vi "Motor control with speed PID.vi"(6 "Motor Connectors":T4={"Enable"="ConnectorB/DIO0", "Input 1"="ConnectorA/DIO1", "Input 2"="ConnectorA/DIO2", "Tach 1"="ConnectorB/DIO8", "Tach 2"="ConnectorB/DIO9"}, 7 "Control":T3={"Motor PWM Control"={"Pulse Lenght DIO3"=10000, "Pulse Period 3"=20000, "Angle"=0}, "stop"=FALSE, "Update Insides Values"=FALSE, "Position Reset"=FALSE}) -> (1 "Speed Output":T5, 2 "Position Output":T6, 3 "Inside values":T7)   [LabVIEW 2013]
uses:
  <vilib>/eio/EIONode/EIONode.xnode
  <vilib>/rvi/eio/common/nirviEmuTemplateMethod_errors.vi
panel:
  in  "Encoder Intputs Motor 3":T1
  in  "Encoder Intputs Motor 2":T1
  out "Incrementation/Decrementation Motor 3":bool
  out "Movement Motor 3":bool
  out "Incrementation/Decrementation Motor 2":bool
  out "Movement Motor 2":bool
  in  "Encoder Intputs Motor 1":T1
  out "Movement Motor 1":bool
  out "Incrementation/Decrementation Motor 1":bool
  in  "Motor Values":T2
  in  "Inside values Motor 3":cluster{"Pulse Lenght":i32, "Angle":i32}
  in  "Inside values Motor 2":cluster{"Pulse Lenght":i32, "Angle":i32}
  in  "Inside values Motor 1":cluster{"Pulse Lenght":i32, "Angle":i32}
  out "Position Reset":bool
  out "Velocity (Counts/Interval)":i32
  out "Degree (absolute)":i32
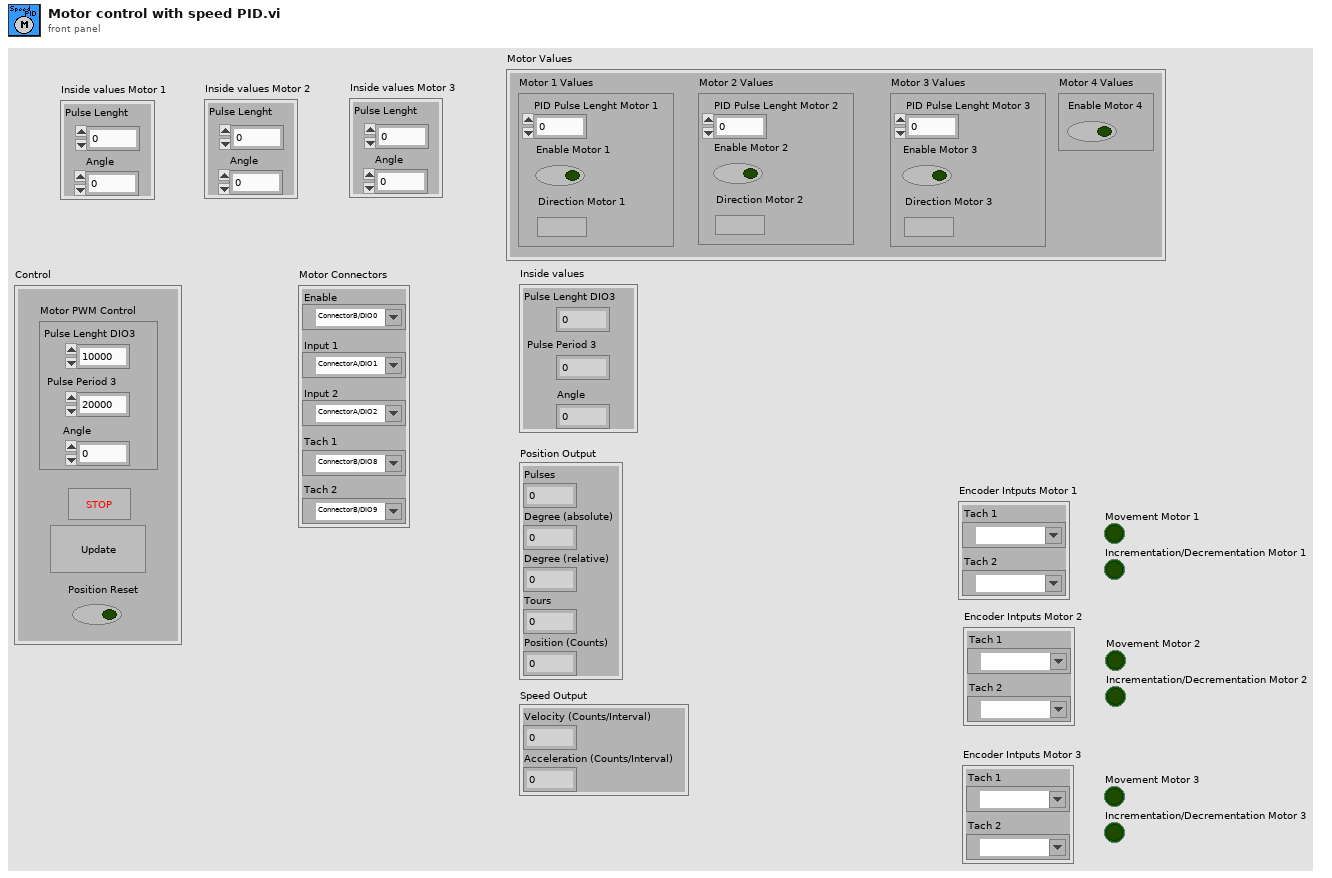
[diagram p1: front panel]
types:
  T1 = cluster{"Tach 2":refnum<k21>, "Tach 1":refnum<k21>}
  T2 = cluster{"Motor 1 Values":cluster{"PID Pulse Lenght Motor 1":i16, "Enable Motor 1":bool, "Direction Motor 1":bool}, "Motor 2 Values":cluster{"PID Pulse Lenght Motor 2":i16, "Enable Motor 2":bool, "Direction Motor 2":bool}, "Motor 3 Values":cluster{"PID Pulse Lenght Motor 3":i16, "Enable Motor 3":bool, "Direction Motor 3":bool}, "Motor 4 Values":cluster{"Enable Motor 4":bool}}
  T3 = cluster{"Motor PWM Control":cluster{"Pulse Lenght DIO3":i32, "Pulse Period 3":i32, "Angle":i32}, "stop":bool, "Update Insides Values":bool, "Position Reset":bool}
  T4 = cluster{"Enable":refnum<k21>, "Input 1":refnum<k21>, "Input 2":refnum<k21>, "Tach 1":refnum<k21>, "Tach 2":refnum<k21>}
  T5 = cluster{"Velocity (Counts/Interval)":i32, "Acceleration (Counts/Interval)":i32}
  T6 = cluster{"Pulses":i32, "Degree (absolute)":i32, "Degree (relative)":i32, "Tours":i32, "Position (Counts)":i32}
  T7 = cluster{"Pulse Lenght DIO3":i32, "Pulse Period 3":i32, "Angle":i32}
  T8 = cluster{"Velocity Interval (uSec)":i32, "I/O Tach 1":bool, "I/O Tach 2":bool, "Position (Counts)":i16, "Boolean Variable 1":bool, "Tick Count(Ticks)":u32, "Position (Counts) 2":i16, "Acceleration (Counts/Interval)":i16, "Velocity (Counts/Interval":i16}
  T9 = cluster{"PID Pulse Lenght Motor 1":i16, "Enable Motor 1":bool, "Direction Motor 1":bool}
  T10 = cluster{"PID Pulse Lenght Motor 2":i16, "Enable Motor 2":bool, "Direction Motor 2":bool}
  T11 = cluster{"PID Pulse Lenght Motor 3":i16, "Enable Motor 3":bool, "Direction Motor 3":bool}
  T12 = cluster{"Tach 1":refnum<k21>, "Tach 2":refnum<k21>}
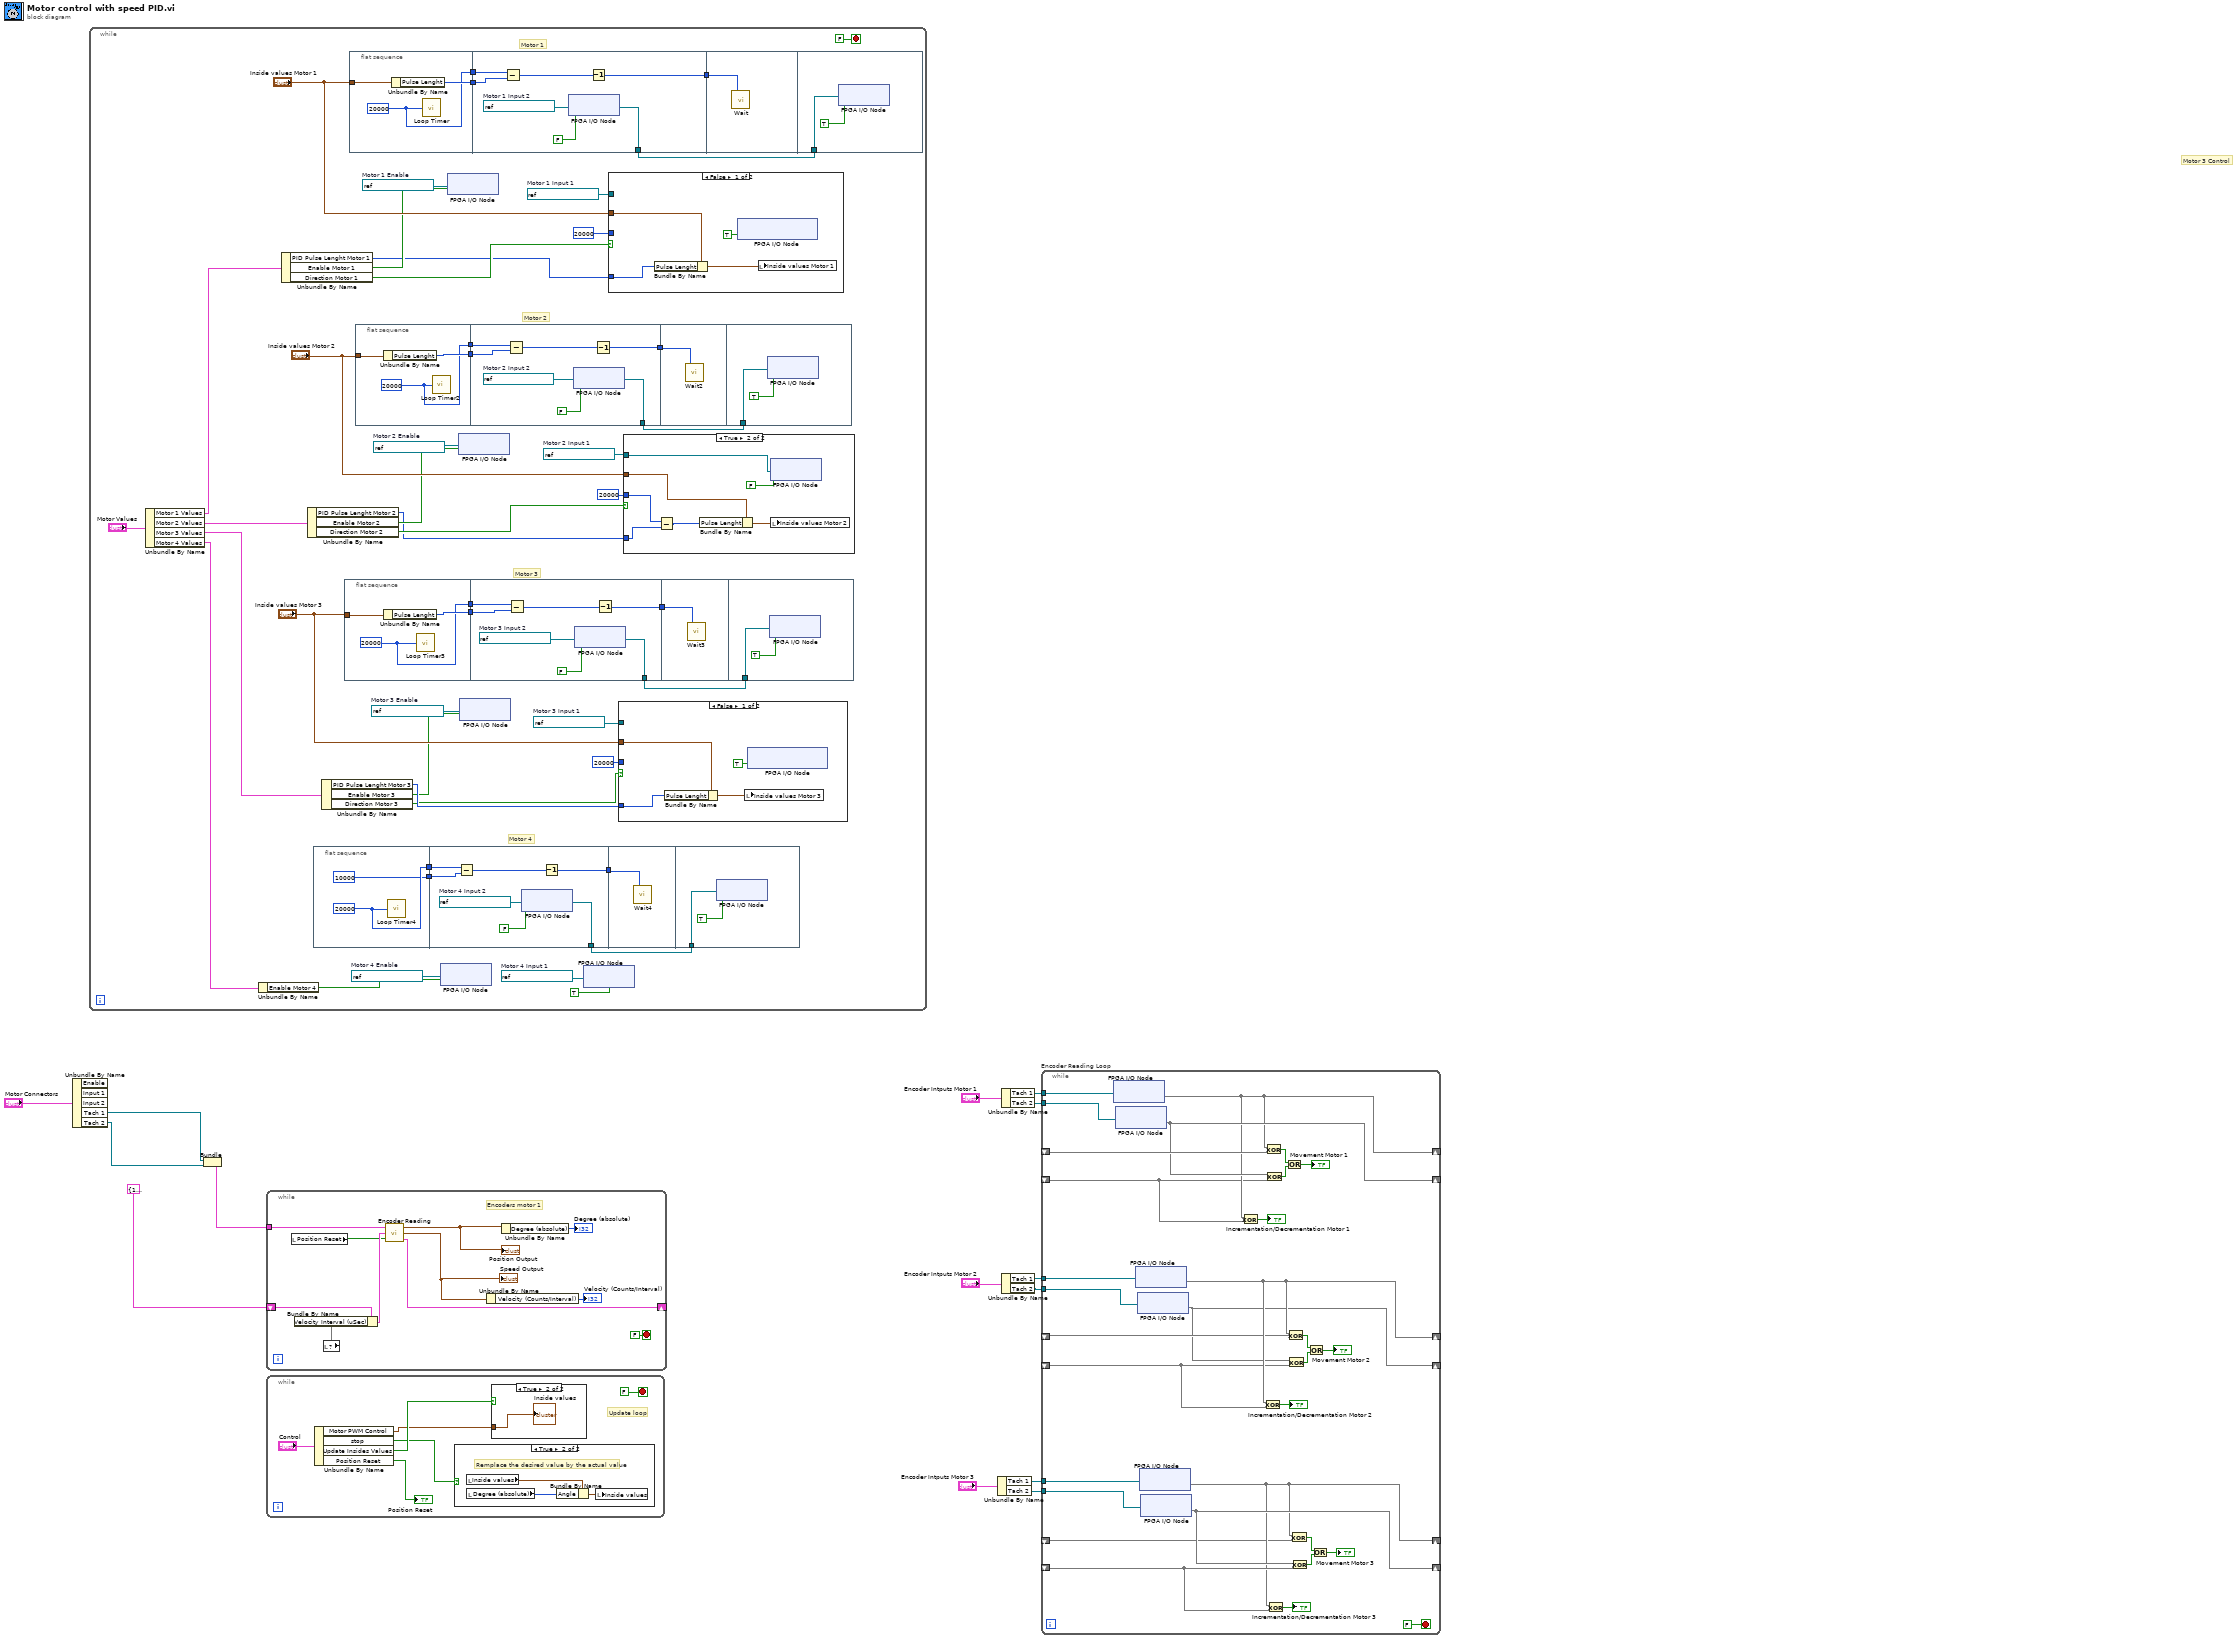
[diagram p0: block diagram]
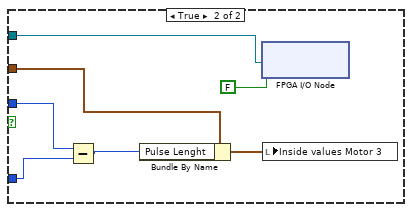
[diagram p2: hidden frame]
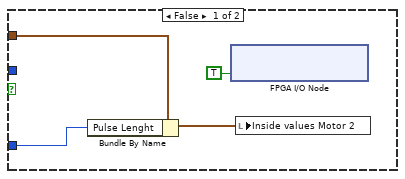
[diagram p3: hidden frame]
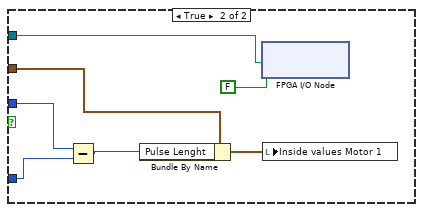
[diagram p4: hidden frame]
diagram:
  # "Motor 3 Control"
  n1 = Unbundle By Name("Motor Connectors") -> ("Tach 1"=w13:refnum<k21>, "Tach 2"=w12:refnum<k21>)  [unwired: 3 out]
  n2 = while {
    stop <- FALSE stop-if-true
    w36 = refnum<k21> "ConnectorA/DIO4"  # Motor 4 Input 1
    w38 = refnum<k21> "ConnectorA/DIO3"  # Motor 4 Enable
    w40 = refnum<k21> "ConnectorA/DIO0"  # Motor 3 Enable
    w39 = refnum<k21> "ConnectorA/DIO1"  # Motor 3 Input 1
    w41 = refnum<k21> "ConnectorB/DIO4"  # Motor 2 Input 1
    w42 = refnum<k21> "ConnectorB/DIO3"  # Motor 2 Enable
    w43 = refnum<k21> "ConnectorB/DIO1"  # Motor 1 Input 1
    w44 = refnum<k21> "ConnectorB/DIO0"  # Motor 1 Enable
    # "Motor 2"
    # "Motor 1"
    # "Motor 3"
    # "Motor 4"
    n3 = Unbundle By Name("Motor Values") -> ("Motor 1 Values"=w28:T9, "Motor 2 Values"=w24:T10, "Motor 3 Values"=w20:T11, "Motor 4 Values"=w16:cluster{"Enable Motor 4":bool})
    n4 = Unbundle By Name(w16) -> ("Enable Motor 4"=w15:bool)
    n5 = Unbundle By Name(w28) -> ("PID Pulse Lenght Motor 1"=w25:i16, "Enable Motor 1"=w27:bool, "Direction Motor 1"=w26:bool)
    n6 = Unbundle By Name(w24) -> ("PID Pulse Lenght Motor 2"=w21:i16, "Enable Motor 2"=w23:bool, "Direction Motor 2"=w22:bool)
    n7 = flat-sequence {
      tunnel: [w63] -> w48
      tunnel: [i16 10000] -> w47
      tunnel: [w70] -> w46
      tunnel: w48 -> [w69]
      tunnel: w47 -> [w68]
      tunnel: [w66] -> w45
      tunnel: w46 -> [w71]
      tunnel: w45 -> [w72]
      frame #0 {
        w63 = i16 20000
        n8 = call "Loop Timer4"("Count(Ticks)"=w63) -> ()  [unwired: 1 out]
      }
      frame #1 {
        w64 = refnum<k21> "ConnectorA/DIO5"  # Motor 4 Input 2
        n9 = Subtract(x=w69, y=w68) -> (x-y=w67:i16)
        n10 = xnode "FPGA I/O Node"("I/O Item"=FALSE ("ConnectorC/DIO7"), "FPGA I/O In"=w64) -> ("FPGA I/O Out"=w66:refnum<k21>)
        n11 = Decrement(x=w67) -> (x-1=w70:i16)
      }
      frame #2 {
        n12 = call "Wait4"("Count(Ticks)"=w71) -> ()  [unwired: 1 out]
      }
      frame #3 {
        n13 = xnode "FPGA I/O Node"("I/O Item"=TRUE ("ConnectorC/DIO7"), "FPGA I/O In"=w72) -> ()  [unwired: 1 out]
      }
    }
    n14 = Unbundle By Name(w20) -> ("PID Pulse Lenght Motor 3"=w19:i16, "Enable Motor 3"=w18:bool, "Direction Motor 3"=w17:bool)
    n15 = flat-sequence {
      tunnel: [w85] -> w52
      tunnel: [w87] -> w51
      tunnel: "Inside values Motor 3" -> [w86]
      tunnel: [w94] -> w50
      tunnel: w52 -> [w93]
      tunnel: w51 -> [w92]
      tunnel: [w90] -> w49
      tunnel: w50 -> [w95]
      tunnel: w49 -> [w96]
      frame #0 {
        w85 = i16 20000
        n16 = Unbundle By Name(w86) -> ("Pulse Lenght"=w87:i32)
        n17 = call "Loop Timer3"("Count(Ticks)"=w85) -> ()  [unwired: 1 out]
      }
      frame #1 {
        w88 = refnum<k21> "ConnectorA/DIO2"  # Motor 3 Input 2
        n18 = Subtract(x=w93, y=w92) -> (x-y=w91:i32)
        n19 = xnode "FPGA I/O Node"("I/O Item"=FALSE ("ConnectorC/DIO7"), "FPGA I/O In"=w88) -> ("FPGA I/O Out"=w90:refnum<k21>)
        n20 = Decrement(x=w91) -> (x-1=w94:i32)
      }
      frame #2 {
        n21 = call "Wait3"("Count(Ticks)"=w95) -> ()  [unwired: 1 out]
      }
      frame #3 {
        n22 = xnode "FPGA I/O Node"("I/O Item"=TRUE ("ConnectorC/DIO7"), "FPGA I/O In"=w96) -> ()  [unwired: 1 out]
      }
    }
    n23 = flat-sequence {
      tunnel: [w133] -> w60
      tunnel: [w135] -> w59
      tunnel: "Inside values Motor 1" -> [w134]
      tunnel: [w142] -> w58
      tunnel: w60 -> [w141]
      tunnel: w59 -> [w140]
      tunnel: [w138] -> w57
      tunnel: w58 -> [w143]
      tunnel: w57 -> [w144]
      frame #0 {
        w133 = i16 20000
        n24 = Unbundle By Name(w134) -> ("Pulse Lenght"=w135:i32)
        n25 = call "Loop Timer"("Count(Ticks)"=w133) -> ()  [unwired: 1 out]
      }
      frame #1 {
        w136 = refnum<k21> "ConnectorB/DIO2"  # Motor 1 Input 2
        n26 = Subtract(x=w141, y=w140) -> (x-y=w139:i32)
        n27 = xnode "FPGA I/O Node"("I/O Item"=FALSE ("ConnectorC/DIO7"), "FPGA I/O In"=w136) -> ("FPGA I/O Out"=w138:refnum<k21>)
        n28 = Decrement(x=w139) -> (x-1=w142:i32)
      }
      frame #2 {
        n29 = call "Wait"("Count(Ticks)"=w143) -> ()  [unwired: 1 out]
      }
      frame #3 {
        n30 = xnode "FPGA I/O Node"("I/O Item"=TRUE ("ConnectorC/DIO7"), "FPGA I/O In"=w144) -> ()  [unwired: 1 out]
      }
    }
    n31 = flat-sequence {
      tunnel: [w109] -> w56
      tunnel: [w111] -> w55
      tunnel: "Inside values Motor 2" -> [w110]
      tunnel: [w118] -> w54
      tunnel: w56 -> [w117]
      tunnel: w55 -> [w116]
      tunnel: [w114] -> w53
      tunnel: w54 -> [w119]
      tunnel: w53 -> [w120]
      frame #0 {
        w109 = i16 20000
        n32 = Unbundle By Name(w110) -> ("Pulse Lenght"=w111:i32)
        n33 = call "Loop Timer2"("Count(Ticks)"=w109) -> ()  [unwired: 1 out]
      }
      frame #1 {
        w112 = refnum<k21> "ConnectorB/DIO5"  # Motor 2 Input 2
        n34 = Subtract(x=w117, y=w116) -> (x-y=w115:i32)
        n35 = xnode "FPGA I/O Node"("I/O Item"=FALSE ("ConnectorC/DIO7"), "FPGA I/O In"=w112) -> ("FPGA I/O Out"=w114:refnum<k21>)
        n36 = Decrement(x=w115) -> (x-1=w118:i32)
      }
      frame #2 {
        n37 = call "Wait2"("Count(Ticks)"=w119) -> ()  [unwired: 1 out]
      }
      frame #3 {
        n38 = xnode "FPGA I/O Node"("I/O Item"=TRUE ("ConnectorC/DIO7"), "FPGA I/O In"=w120) -> ()  [unwired: 1 out]
      }
    }
    n39 = xnode "FPGA I/O Node"("I/O Item"=w15, "FPGA I/O In"=w38) -> ()  [unwired: 1 out]
    n40 = xnode "FPGA I/O Node"("I/O Item"=w27, "FPGA I/O In"=w44) -> ()  [unwired: 1 out]
    n41 = xnode "FPGA I/O Node"("I/O Item"=w23, "FPGA I/O In"=w42) -> ()  [unwired: 1 out]
    n42 = xnode "FPGA I/O Node"("I/O Item"=w18, "FPGA I/O In"=w40) -> ()  [unwired: 1 out]
    n43 = xnode "FPGA I/O Node"("I/O Item"=TRUE ("ConnectorC/DIO7"), "FPGA I/O In"=w36) -> ()  [unwired: 1 out]
    n44 = case shown="False" w26 {
      tunnel: w25 -> [w123 w131]
      tunnel: "Inside values Motor 1" -> [w122 w128]
      tunnel: i16 20000 -> [_ w132]
      tunnel: w43 -> [_ w126]
      frame False {
        n45 = Bundle By Name(cluster=w122, "Pulse Lenght"=w123) -> (w124:cluster{"Pulse Lenght":i32, "Angle":i32})
        n46 = xnode "FPGA I/O Node"("ConnectorB/DIO1"=TRUE ("ConnectorC/DIO7")) -> ()  [unwired: 1 in, 1 out]
        n47 = local write "Inside values Motor 1"(w124) -> ()
      }
      frame True {
        n48 = Subtract(x=w132, y=w131) -> (x-y=w129:i16)
        n49 = Bundle By Name(cluster=w128, "Pulse Lenght"=w129) -> (w130:cluster{"Pulse Lenght":i32, "Angle":i32})
        n50 = xnode "FPGA I/O Node"("I/O Item"=FALSE ("ConnectorC/DIO7"), "FPGA I/O In"=w126) -> ()  [unwired: 1 out]
        n51 = local write "Inside values Motor 1"(w130) -> ()
      }
    }
    n52 = case shown="False" w17 {
      tunnel: w19 -> [w75 w83]
      tunnel: "Inside values Motor 3" -> [w74 w80]
      tunnel: 20000 ("Pulse Period 3") -> [_ w84]
      tunnel: w39 -> [_ w78]
      frame False {
        n53 = Bundle By Name(cluster=w74, "Pulse Lenght"=w75) -> (w76:cluster{"Pulse Lenght":i32, "Angle":i32})
        n54 = local write "Inside values Motor 3"(w76) -> ()
        n55 = xnode "FPGA I/O Node"("ConnectorB/DIO1"=TRUE ("ConnectorC/DIO7")) -> ()  [unwired: 1 in, 1 out]
      }
      frame True {
        n56 = Subtract(x=w84, y=w83) -> (x-y=w81:i32)
        n57 = Bundle By Name(cluster=w80, "Pulse Lenght"=w81) -> (w82:cluster{"Pulse Lenght":i32, "Angle":i32})
        n58 = xnode "FPGA I/O Node"("I/O Item"=FALSE ("ConnectorC/DIO7"), "FPGA I/O In"=w78) -> ()  [unwired: 1 out]
        n59 = local write "Inside values Motor 3"(w82) -> ()
      }
    }
    n60 = case shown="True" w22 {
      tunnel: w21 -> [w99 w107]
      tunnel: "Inside values Motor 2" -> [w98 w104]
      tunnel: 20000 ("Pulse Period 3") -> [_ w108]
      tunnel: w41 -> [_ w102]
      frame False {
        n61 = Bundle By Name(cluster=w98, "Pulse Lenght"=w99) -> (w100:cluster{"Pulse Lenght":i32, "Angle":i32})
        n62 = xnode "FPGA I/O Node"("ConnectorB/DIO1"=TRUE ("ConnectorC/DIO7")) -> ()  [unwired: 1 in, 1 out]
        n63 = local write "Inside values Motor 2"(w100) -> ()
      }
      frame True {
        n64 = Subtract(x=w108, y=w107) -> (x-y=w105:i32)
        n65 = Bundle By Name(cluster=w104, "Pulse Lenght"=w105) -> (w106:cluster{"Pulse Lenght":i32, "Angle":i32})
        n66 = xnode "FPGA I/O Node"("I/O Item"=FALSE ("ConnectorC/DIO7"), "FPGA I/O In"=w102) -> ()  [unwired: 1 out]
        n67 = local write "Inside values Motor 2"(w106) -> ()
      }
    }
  }
  n68 = Bundle("Tach 1"=w13, "Tach 2"=w12) -> (w11:T12)  [unwired: 1 in]
  n69 = while {
    shift-right: [w154] -> _
    shift-left: T8 {"Velocity Interval (uSec)"=1000000, "I/O Tach 1"=FALSE, "I/O Tach 2"=FALSE, "Position (Counts)"=0, "Boolean Variable 1"=FALSE, "Tick Count(Ticks)"=0, "Position (Counts) 2"=0, "Acceleration (Counts/Interval)"=0, "Velocity (Counts/Interval"=0} ("Values") -> [w149]
    tunnel: w11 -> [w155]
    stop <- FALSE stop-if-true
    # "Encoders motor 1"
    n70 = local read "Position Reset"() -> (w147:bool)
    n71 = local read item#-1() -> (w146)
    n72 = Bundle By Name(cluster=w149, "Velocity Interval (uSec)"=w146) -> (w148:T8)
    n73 = call "Encoder Reading.vi"("Position Reset"=w147, "Values"=w148, "Encoder Intputs"=w155) -> ("output cluster"=w154:T8, "Speed Output"=w150:T5, "Position Output"=w151:T6)
    "Position Output" <- w151
    "Speed Output" <- w150
    n74 = Unbundle By Name(w150) -> ("Velocity (Counts/Interval)"=→"Velocity (Counts/Interval)":i32)
    n75 = Unbundle By Name(w151) -> ("Degree (absolute)"=→"Degree (absolute)":i32)
  }
  n76 = while {
    stop <- FALSE stop-if-true
    # "Update loop"
    n77 = Unbundle By Name("Control") -> ("Motor PWM Control"=w158:T7, "stop"=w159:bool, "Update Insides Values"=w160:bool, "Position Reset"=→"Position Reset":bool)
    n78 = case shown="True" w159 {
      frame False {
      }
      frame True {
        # "Remplace the desired value by the actual value"
        n79 = local read "Inside values"() -> (w165:T7)
        n80 = local read "Degree (absolute)"() -> (w164:i32)
        n81 = Bundle By Name(cluster=w165, "Angle"=w164) -> (w163:T7)
        n82 = local write "Inside values"(w163) -> ()
      }
    }
    n83 = case shown="True" w160 {
      tunnel: w158 -> [_ w166]
      frame False {
      }
      frame True {
        "Inside values" <- w166
      }
    }
  }
  n84 = Unbundle By Name("Encoder Intputs Motor 3") -> ("Tach 1"=w2:refnum<k21>, "Tach 2"=w1:refnum<k21>)
  n85 = Unbundle By Name("Encoder Intputs Motor 1") -> ("Tach 1"=w8:refnum<k21>, "Tach 2"=w7:refnum<k21>)
  n86 = Unbundle By Name("Encoder Intputs Motor 2") -> ("Tach 1"=w4:refnum<k21>, "Tach 2"=w3:refnum<k21>)
  n87 = while "Encoder Reading Loop" {
    tunnel: w8 -> [w197]
    tunnel: w7 -> [w196]
    shift-right: [w190] -> _
    shift-left: _ -> [w193]
    shift-right: [w192] -> _
    shift-left: _ -> [w189]
    shift-right: [w182] -> _
    shift-left: _ -> [w181]
    shift-right: [w179] -> _
    shift-left: _ -> [w180]
    shift-right: [w172] -> _
    shift-left: _ -> [w171]
    shift-right: [w173] -> _
    shift-left: _ -> [w174]
    tunnel: w4 -> [w170]
    tunnel: w3 -> [w169]
    tunnel: w2 -> [w168]
    tunnel: w1 -> [w167]
    stop <- FALSE stop-if-true
    n88 = xnode "FPGA I/O Node"("FPGA I/O In"=w197) -> ("I/O Item"=w190)  [unwired: 1 out]
    n89 = xnode "FPGA I/O Node"("FPGA I/O In"=w196) -> ("I/O Item"=w192)  [unwired: 1 out]
    n90 = xnode "FPGA I/O Node"("FPGA I/O In"=w170) -> ("I/O Item"=w182)  [unwired: 1 out]
    n91 = xnode "FPGA I/O Node"("FPGA I/O In"=w169) -> ("I/O Item"=w179)  [unwired: 1 out]
    n92 = xnode "FPGA I/O Node"("FPGA I/O In"=w168) -> ("I/O Item"=w172)  [unwired: 1 out]
    n93 = xnode "FPGA I/O Node"("FPGA I/O In"=w167) -> ("I/O Item"=w173)  [unwired: 1 out]
    n94 = Exclusive Or(1:w189, 2:w190) -> (0:→"Incrementation/Decrementation Motor 1":bool)
    n95 = Exclusive Or(1:w180, 2:w182) -> (0:→"Incrementation/Decrementation Motor 2":bool)
    n96 = Exclusive Or(1:w193, 2:w190) -> (0:w194:bool)
    n97 = Exclusive Or(1:w189, 2:w192) -> (0:w195:bool)
    n98 = Exclusive Or(1:w174, 2:w172) -> (0:→"Incrementation/Decrementation Motor 3":bool)
    n99 = Or(x=w194, y=w195) -> (x .or. y?=→"Movement Motor 1":bool)
    n100 = Exclusive Or(1:w181, 2:w182) -> (0:w185:bool)
    n101 = Exclusive Or(1:w180, 2:w179) -> (0:w186:bool)
    n102 = Exclusive Or(1:w171, 2:w172) -> (0:w177:bool)
    n103 = Exclusive Or(1:w174, 2:w173) -> (0:w178:bool)
    n104 = Or(x=w185, y=w186) -> (x .or. y?=→"Movement Motor 2":bool)
    n105 = Or(x=w177, y=w178) -> (x .or. y?=→"Movement Motor 3":bool)
  }
